vi "RichToFlatcif_manager_QuerySystemStatusRequest.vi"(5 "OutputClusterType":T1, 11 "InputCluster":T16) -> (3 "OutputCluster":T1)   [LabVIEW 2021, in "CIF_Manager_client.lvlib"]
uses:
  CIF_Manager_client.lvlib
  cif_manager_QuerySystemStatusRequest.ctl
  cif_manager_PluginStatus.ctl
  cif_management_common_PluginStatusData.ctl
  cif_management_common_PluginStatusData_PluginState.ctl
  cif_management_common_TimingStatistics.ctl
  cif_common_TimingStats.ctl
  cif_management_common_FifoStatistics.ctl
  cif_management_common_Error.ctl
  cif_management_common_MonitorDoubles.ctl
  cif_management_common_MonitorU64.ctl
  cif_management_common_MonitorI64.ctl
  cif_management_common_Channels.ctl
  cif_management_common_Channel.ctl
  cif_management_common_ChannelDirection.ctl
  cif_management_common_ChannelPattern.ctl
  cif_manager_QuerySystemStatusRequest_Flat.ctl
  cif_manager_PluginStatus_Flat.ctl
  cif_management_common_PluginStatusData_Flat.ctl
  cif_management_common_TimingStatistics_Flat.ctl
  cif_common_TimingStats_Flat.ctl
  cif_management_common_FifoStatistics_Flat.ctl
  cif_management_common_Error_Flat.ctl
  cif_management_common_MonitorDoubles_Flat.ctl
  cif_management_common_MonitorU64_Flat.ctl
  cif_management_common_MonitorI64_Flat.ctl
  cif_management_common_Channels_Flat.ctl
  cif_management_common_Channel_Flat.ctl
  RichToFlatcif_management_common_PluginStatusData.vi
  RichToFlatcif_management_common_Channels.vi
  RichToFlatcif_management_common_TimingStatistics.vi
  RichToFlatcif_management_common_FifoStatistics.vi
  RichToFlatcif_management_common_Error.vi
  RichToFlatcif_management_common_MonitorDoubles.vi
  RichToFlatcif_management_common_MonitorU64.vi
  RichToFlatcif_management_common_MonitorI64.vi
  RichToFlatcif_management_common_Channel.vi
  RichToFlatcif_common_TimingStats.vi
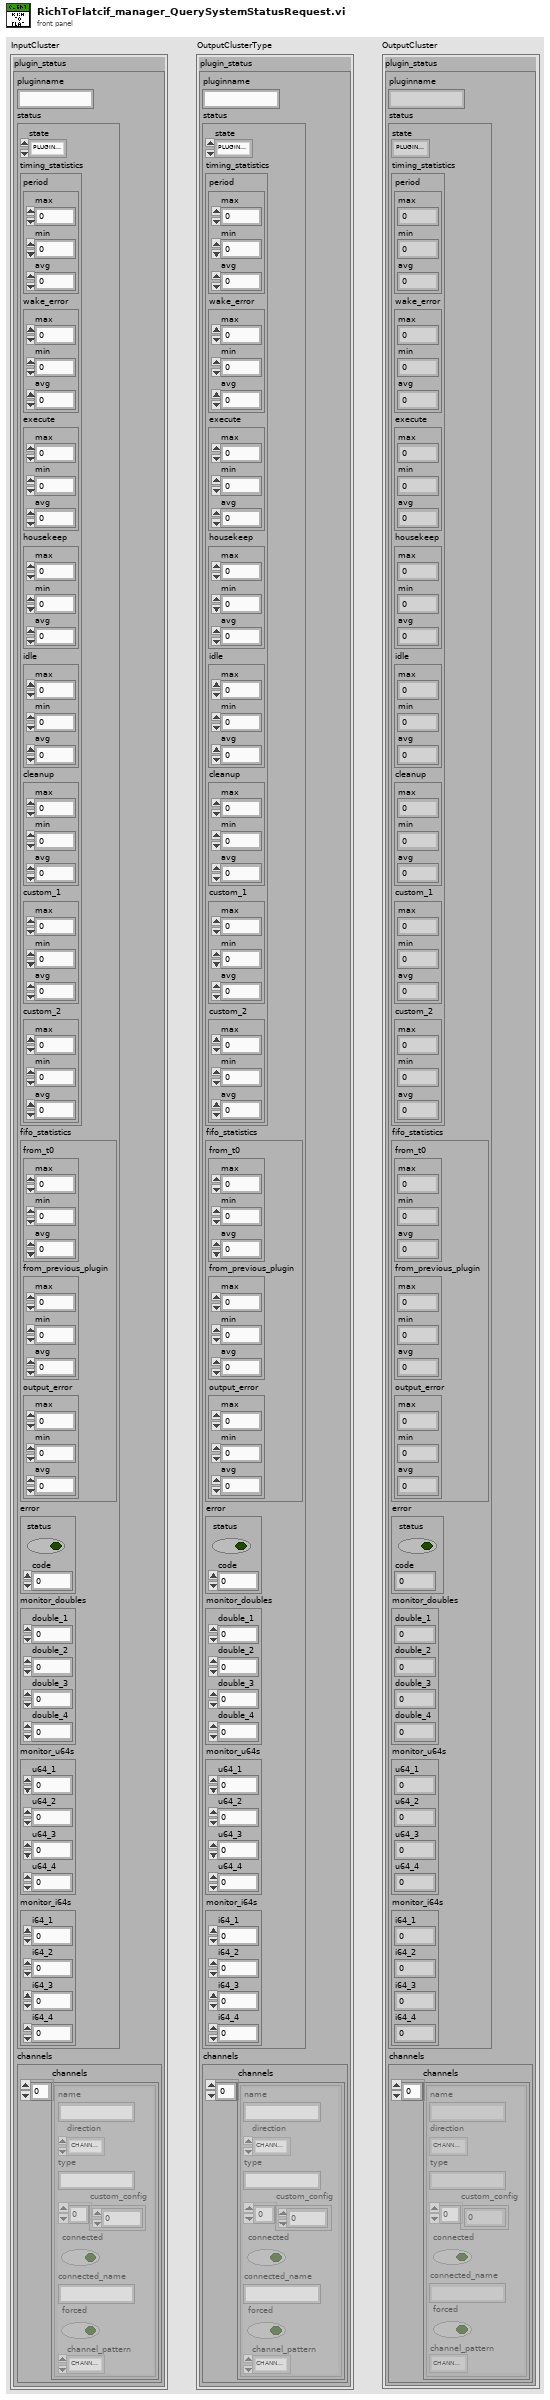
[diagram p1: front panel]
types:
  T1 = typedef "CIF_Manager_client.lvlib/cif_manager_QuerySystemStatusRequest_Flat.ctl" = cluster{"plugin_status":T2}
  T2 = typedef "CIF_Manager_client.lvlib/cif_manager_PluginStatus_Flat.ctl" = cluster{"pluginname":string, "status":T3, "channels":T12}
  T3 = typedef "CIF_Manager_client.lvlib/cif_management_common_PluginStatusData_Flat.ctl" = cluster{"state":T4, "timing_statistics":T5, "fifo_statistics":T7, "error":T8, "monitor_doubles":T9, "monitor_u64s":T10, "monitor_i64s":T11}
  T4 = typedef "CIF_Manager_client.lvlib/cif_management_common_PluginStatusData_PluginState.ctl" = enum32{"PLUGINSTATE_UNKNOWN", "PLUGINSTATE_CREATING", "PLUGINSTATE_LISTENING", "PLUGINSTATE_RUNNING", "PLUGINSTATE_CLEANINGUP", "PLUGINSTATE_DESTROYING", "PLUGINSTATE_PREPARED", "PLUGINSTATE_FTE_RUN"}
  T5 = typedef "CIF_Manager_client.lvlib/cif_management_common_TimingStatistics_Flat.ctl" = cluster{"period":T6, "wake_error":T6, "execute":T6, "housekeep":T6, "idle":T6, "cleanup":T6, "custom_1":T6, "custom_2":T6}
  T6 = typedef "CIF_Manager_client.lvlib/cif_common_TimingStats_Flat.ctl" = cluster{"max":i64, "min":i64, "avg":dbl}
  T7 = typedef "CIF_Manager_client.lvlib/cif_management_common_FifoStatistics_Flat.ctl" = cluster{"from_t0":T6, "from_previous_plugin":T6, "output_error":T6}
  T8 = typedef "CIF_Manager_client.lvlib/cif_management_common_Error_Flat.ctl" = cluster{"status":bool, "code":i32}
  T9 = typedef "CIF_Manager_client.lvlib/cif_management_common_MonitorDoubles_Flat.ctl" = cluster{"double_1":dbl, "double_2":dbl, "double_3":dbl, "double_4":dbl}
  T10 = typedef "CIF_Manager_client.lvlib/cif_management_common_MonitorU64_Flat.ctl" = cluster{"u64_1":u64, "u64_2":u64, "u64_3":u64, "u64_4":u64}
  T11 = typedef "CIF_Manager_client.lvlib/cif_management_common_MonitorI64_Flat.ctl" = cluster{"i64_1":i64, "i64_2":i64, "i64_3":i64, "i64_4":i64}
  T12 = typedef "CIF_Manager_client.lvlib/cif_management_common_Channels_Flat.ctl" = cluster{"channels":T13[]}
  T13 = typedef "CIF_Manager_client.lvlib/cif_management_common_Channel_Flat.ctl" = cluster{"name":string, "direction":T14, "type":string, "custom_config":u8[], "connected":bool, "connected_name":string, "forced":bool, "channel_pattern":T15}
  T14 = typedef "CIF_Manager_client.lvlib/cif_management_common_ChannelDirection.ctl" = enum32{"CHANNELDIRECTION_UNKNOWN", "CHANNELDIRECTION_PUBLISHER", "CHANNELDIRECTION_SUBSCRIBER"}
  T15 = typedef "CIF_Manager_client.lvlib/cif_management_common_ChannelPattern.ctl" = enum32{"CHANNELPATTERN_UNKNOWN", "CHANNELPATTERN_TAG", "CHANNELPATTERN_FIFO", "CHANNELPATTERN_MULTIFIFO", "CHANNELPATTERN_BACKPRESSUREFIFO"}
  T16 = typedef "CIF_Manager_client.lvlib/cif_manager_QuerySystemStatusRequest.ctl" = cluster{"plugin_status":T17}
  T17 = typedef "CIF_Manager_client.lvlib/cif_manager_PluginStatus.ctl" = cluster{"pluginname":string, "status":T18, "channels":T26}
  T18 = typedef "CIF_Manager_client.lvlib/cif_management_common_PluginStatusData.ctl" = cluster{"state":T4, "timing_statistics":T19, "fifo_statistics":T21, "error":T22, "monitor_doubles":T23, "monitor_u64s":T24, "monitor_i64s":T25}
  T19 = typedef "CIF_Manager_client.lvlib/cif_management_common_TimingStatistics.ctl" = cluster{"period":T20, "wake_error":T20, "execute":T20, "housekeep":T20, "idle":T20, "cleanup":T20, "custom_1":T20, "custom_2":T20}
  T20 = typedef "CIF_Manager_client.lvlib/cif_common_TimingStats.ctl" = cluster{"max":i64, "min":i64, "avg":dbl}
  T21 = typedef "CIF_Manager_client.lvlib/cif_management_common_FifoStatistics.ctl" = cluster{"from_t0":T20, "from_previous_plugin":T20, "output_error":T20}
  T22 = typedef "CIF_Manager_client.lvlib/cif_management_common_Error.ctl" = cluster{"status":bool, "code":i32}
  T23 = typedef "CIF_Manager_client.lvlib/cif_management_common_MonitorDoubles.ctl" = cluster{"double_1":dbl, "double_2":dbl, "double_3":dbl, "double_4":dbl}
  T24 = typedef "CIF_Manager_client.lvlib/cif_management_common_MonitorU64.ctl" = cluster{"u64_1":u64, "u64_2":u64, "u64_3":u64, "u64_4":u64}
  T25 = typedef "CIF_Manager_client.lvlib/cif_management_common_MonitorI64.ctl" = cluster{"i64_1":i64, "i64_2":i64, "i64_3":i64, "i64_4":i64}
  T26 = typedef "CIF_Manager_client.lvlib/cif_management_common_Channels.ctl" = cluster{"channels":T27[]}
  T27 = typedef "CIF_Manager_client.lvlib/cif_management_common_Channel.ctl" = cluster{"name":string, "direction":T14, "type":string, "custom_config":u8[], "connected":bool, "connected_name":string, "forced":bool, "channel_pattern":T15}
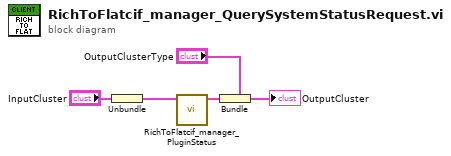
[diagram p0: block diagram]
diagram:
  n1 = Unbundle "Unbundle"("InputCluster") -> ("plugin_status"=w2:T17)
  n2 = call "RichToFlatcif_manager_PluginStatus.vi"("InputCluster"=w2) -> ("OutputCluster"=w1:T2)  [unwired: 10 in]
  n3 = Bundle "Bundle"(cluster="OutputClusterType", "plugin_status"=w1) -> (→"OutputCluster":T1)
